vi "DSF.Engine.Pointer.Status.Builder.State.New.vi"(8 "error in (no error)":errorcluster, 10 "count (1)":u64=1, 11 "Builder State Pointer type":refnum<class "DSF.Engine.Pointer.Status.Builder.State.lvclass">) -> (0 "error out":errorcluster, 3 "Builder State Pointer":refnum<class "DSF.Engine.Pointer.Status.Builder.State.lvclass">)   [LabVIEW 2016, in "DSF.Engine.lvlib" / "DSF.Engine.Pointer.Status.Builder.State.lvclass"]
uses:
  Pointer/DSF.Engine.Pointer.Status.Builder.State.lvclass
  C:/Git/Sourcetree/DSF/Source/Submodules/Memory/Source/Classes/Pointer/Memory.Pointer.lvclass
  Submodules/Memory/Source/Classes/Pointer/Memory.Pointer.New.1B.vi
  Submodules/Memory/Source/Classes/Pointer/Memory.Pointer.Allocate.vi
  Submodules/Memory/Source/Classes/Pointer/Memory.Pointer.lvclass
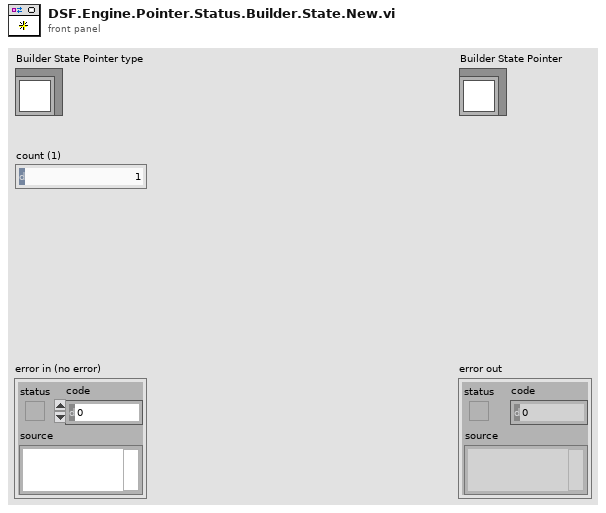
[diagram p1: front panel]
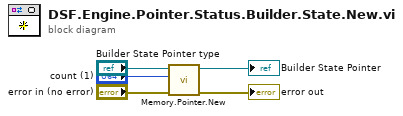
[diagram p0: block diagram]
diagram:
  n1 = call-poly "Memory.Pointer.New.vi"("error in (no error)"="error in (no error)", "count (1)"="count (1)", "pointer type"="Builder State Pointer type") -> ("error out"=→"error out":errorcluster, "pointer out"=→"Builder State Pointer":refnum<class "DSF.Engine.Pointer.Status.Builder.State.lvclass">)  [unwired: 7 in]
